vi "Destroy.vi"(8 "error in (no error)":errorcluster, 11 "Image Distorter in":refnum<class "Image Distorter.lvclass">) -> (0 "error out":errorcluster)   [LabVIEW 2020, in "image.lvlib" / "Image Distorter.lvclass"]
doc: "Destroy the Image Distorter and clear up any associated resources."
uses:
  Image Distorter.lvclass
  Image Distorter.lvclass/Image Distorter.ctl
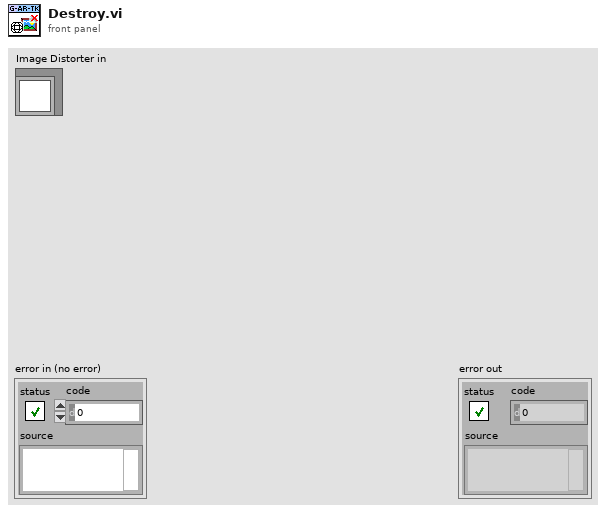
[diagram p1: front panel]
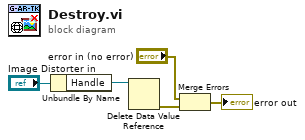
[diagram p0: block diagram]
diagram:
  n1 = Unbundle By Name("Image Distorter in") -> ("Handle"=w3:refnum<data-value>)
  n2 = Delete Data Value Reference(data value reference=w3) -> (error out=w1:errorcluster)  [unwired: 1 in, 1 out]
  n3 = Merge Errors("error in (no error)", w1) -> (→"error out":errorcluster)
